vi "Read QMH Payload.vi"(8 "error in (no error)":errorcluster, 11 "QMHMessagePayload in":refnum<class "QMHMessagePayload.lvclass">) -> (0 "error out":errorcluster, 2 "QMH Payload":variant, 3 "QMHMessagePayload out":refnum<class "QMHMessagePayload.lvclass">)   [LabVIEW 2016, in "QMHMessagePayload.lvclass"]
uses:
  QMHMessagePayload.lvclass
  QMHMessagePayload.lvclass/QMHMessagePayload.ctl
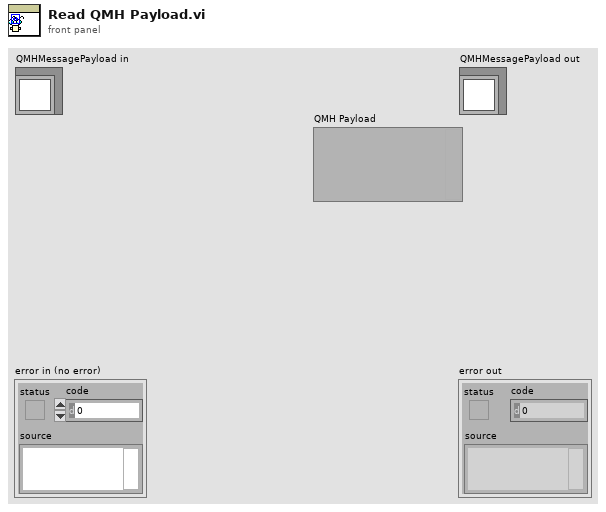
[diagram p1: front panel]
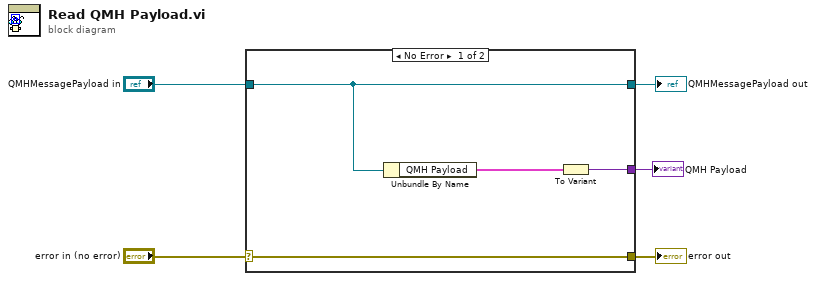
[diagram p0: block diagram]
diagram:
  n1 = case shown="No Error" "error in (no error)" {
    selector: "error in (no error)" -> [w9 w10]
    tunnel: [w9 w10] -> w4
    tunnel: [w8 w11] -> w2
    tunnel: "QMHMessagePayload in" -> [w8 w11]
    tunnel: [w6 _] -> w1
    frame No Error {
      n2 = Unbundle By Name(w8) -> ("QMH Payload"=w7:cluster{"State":enum16{""}, "Data":variant})
      n3 = To Variant(anything=w7) -> (Variant=w6:variant)
    }
    frame Error {
    }
  }
  "error out" <- w4
  "QMHMessagePayload out" <- w2
  "QMH Payload" <- w1
